vi "Google Earth - initialise.vi"(8 "error in (no error)":errorcluster, 11 "EARTHLib.IApplicationGE":refnum<k7>) -> (0 "error out":errorcluster, 2 "IsInitialized":i32, 3 "Refnum Out":refnum<k7>)   [LabVIEW 2009]
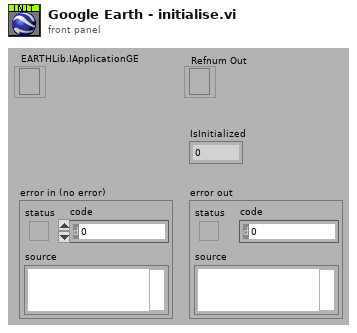
[diagram p1: front panel]
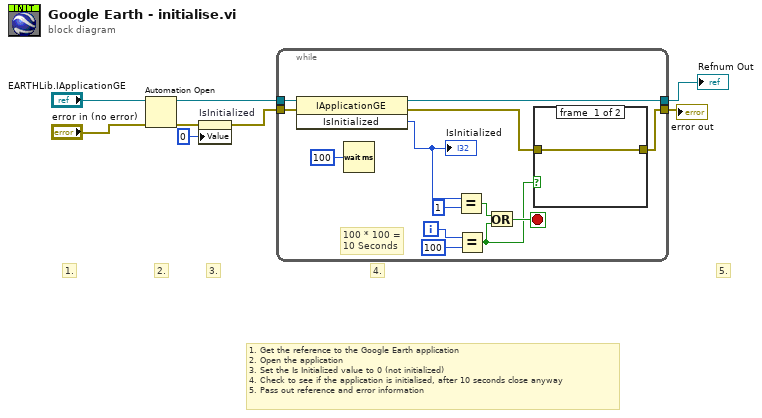
[diagram p0: block diagram]
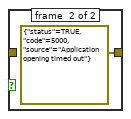
[diagram p2: hidden frame]
diagram:
  # "1. Get the reference to the Google Earth application\n2. Open the application\n3. Set the Is Initialized value to 0 (not initialized)\n4. Check to see if the application is initialised, after 10 seconds close anyway\n5. Pass out reference and error information"
  # "5."
  # "4."
  # "3."
  # "2."
  # "1."
  n1 = Automation Open(error in (no error)="error in (no error)", Automation Refnum="EARTHLib.IApplicationGE") -> (Automation Refnum=w6:refnum<k7>, error out=w5:errorcluster)  [unwired: 2 in]
  n2 = property on="IsInitialized" class="DigNum (strict)"(error in=w5, "Value"=0 ("IsInitialized")) -> (error out=w4:errorcluster)  [unwired: 1 in, 1 out]
  n3 = while {
    tunnel: [w9] -> w1
    tunnel: [w21] -> w8
    tunnel: w6 -> [w20]
    tunnel: w4 -> [w19]
    i -> [w13]
    stop <- w14 stop-if-true
    # "100 * 100 =\n10 Seconds"
    n4 = invoke class="IApplicationGE" method="IsInitialized"(reference=w20, error in=w19) -> (reference out=w21:refnum<k7>, error out=w10:errorcluster, "IsInitialized"=w18:i32)  [unwired: 1 in]
    "IsInitialized" <- w18
    n5 = Wait (ms)(milliseconds to wait=u32 100) -> ()  [unwired: 1 out]
    n6 = Equal?(x=w18, y=1) -> (x = y?=w15:bool)
    n7 = Equal?(x=w13, y=100) -> (x = y?=w11:bool)
    n8 = Or(x=w15, y=w11) -> (x .or. y?=w14:bool)
    n9 = case shown="True" w11 {
      tunnel: w10 -> [w22 _]
      tunnel: [w22 errorcluster {"status"=TRUE, "code"=5000, "source"="Application opening timed out"} ("error out")] -> w9
      frame #0 {
      }
      frame #1 {
      }
    }
  }
  "Refnum Out" <- w8
  "error out" <- w1
